vi "Calculator-V1.0.vi"() -> ()   [LabVIEW 2014]
panel:
  out "?":string
  out "?":string
  out "?":string
  out "?":string
  out "output cluster":cluster{dbl, dbl, dbl, dbl}
  in  "y":dbl
  in  "x":dbl
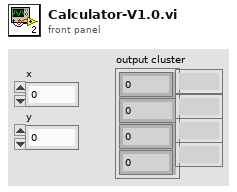
[diagram p1: front panel]
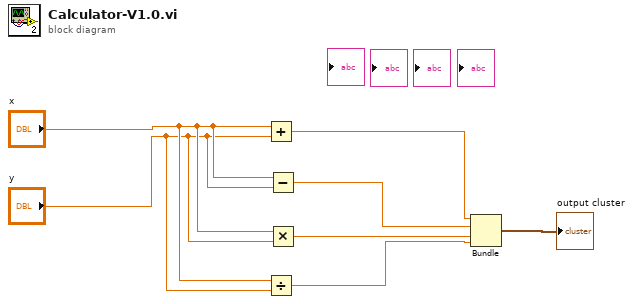
[diagram p0: block diagram]
diagram:
  n1 = Add(x="x", y="y") -> (x+y=w5:dbl)
  n2 = Divide(x="x", y="y") -> (x/y=w2:dbl)
  n3 = Subtract(x="x", y="y") -> (x-y=w4:dbl)
  n4 = Multiply(x="x", y="y") -> (x*y=w3:dbl)
  n5 = Bundle(w5, w4, w3, w2) -> (→"output cluster":cluster{dbl, dbl, dbl, dbl})  [unwired: 1 in]
